vi "Visualize Puzzle.vi"(7 "Jump Points":set{T2}(c389), 10 "Direction Planes":T1[][][](array[typedef]), 11 "Wall Array":T1[][](array[typedef])) -> (3 "Array out":T1[][](array[typedef]))   [LabVIEW 2020]
uses:
  RB ENUM_Position ID.ctl
  Cluster _Point Location.ctl
  038fd235-bb71-4006-9680-315b02cd736b.vi
  <vilib>/Comparison/Equal/Equal Functor/Equal Functor.lvclass
panel:
  out "colum":i32
  out "row":i32
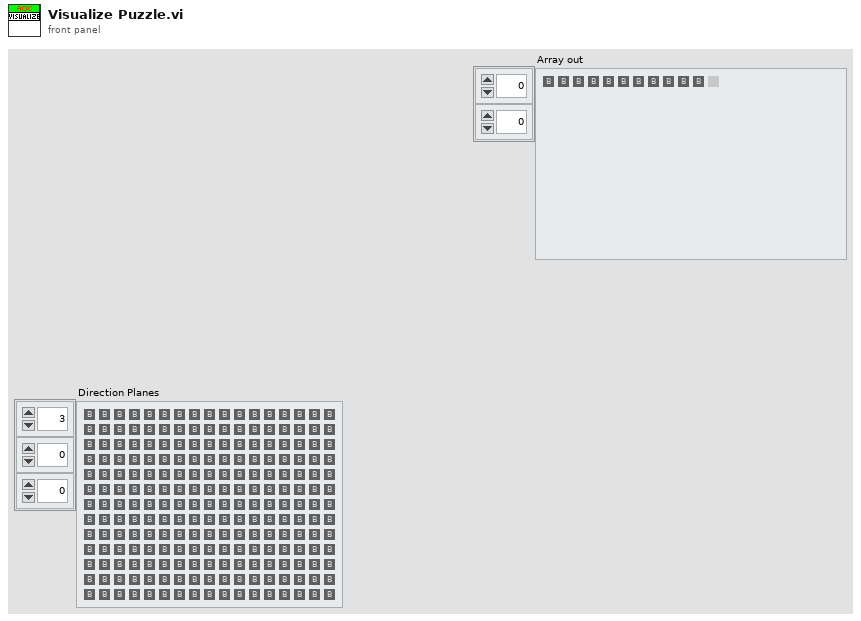
[diagram p1: front panel]
types:
  T1 = typedef "RB ENUM_Position ID.ctl" = enum32{"Blank", "Wall", "UP", "Down", "Left", "Right", "Two", "Three", "Four", "Spot"}
  T2 = typedef "Cluster _Point Location.ctl" = cluster{"X col":i32, "Y row":i32}
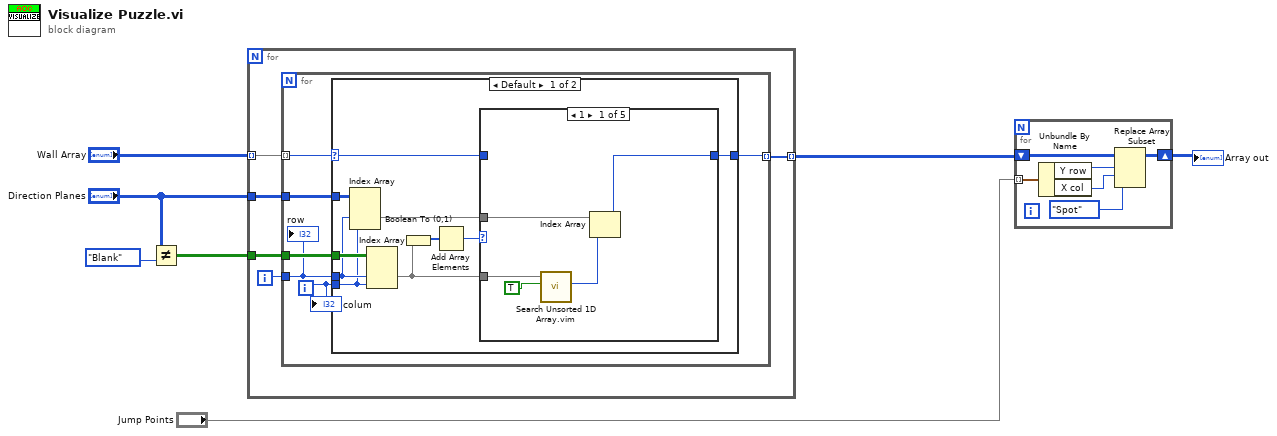
[diagram p0: block diagram]
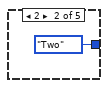
[diagram p2: hidden frame]
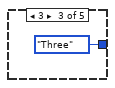
[diagram p3: hidden frame]
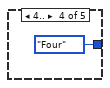
[diagram p4: hidden frame]
diagram:
  n1 = Not Equal?(x="Direction Planes", y=RB_ENUM_Position_ID."Blank" ("Position")) -> (x != y?=w1:bool[][][])
  n2 = for {
    tunnel: "Wall Array" -> [w12] mode=indexing
    tunnel: [w11] -> w4 mode=indexing
    tunnel: "Direction Planes" -> [w10]
    tunnel: w1 -> [w9]
    i -> [w8]
    n3 = for {
      tunnel: w12 -> [w18] mode=indexing
      tunnel: [w17] -> w11 mode=indexing
      tunnel: w10 -> [w13]
      tunnel: w9 -> [w16]
      tunnel: w8 -> [w15]
      i -> [w14]
      n4 = case shown="Default" w18 {
        selector: w18 -> [w24 w38]
        tunnel: [w23 w38] -> w17
        tunnel: w16 -> [w28 _]
        tunnel: w15 -> [w26 _]
        tunnel: w14 -> [w25 _]
        tunnel: w13 -> [w27 _]
        frame Default {
          n5 = Index Array(array=w27, index (dim 1)=w26, index (dim 2)=w25) -> (element=w22:T1[])  [unwired: 1 in]
          n6 = Index Array(array=w28, index (dim 1)=w26, index (dim 2)=w25) -> (element=w21:bool[])  [unwired: 1 in]
          n7 = Boolean To (0,1)(Boolean=w21) -> (0, 1=w19:i16[])
          n8 = Add Array Elements(numeric array=w19) -> (sum=w20:i16)
          n9 = case shown="1" w20 {
            tunnel: w24 -> [_ _ _ _ w37]
            tunnel: [w30 RB_ENUM_Position_ID."Two" ("Position") RB_ENUM_Position_ID."Three" ("Position") RB_ENUM_Position_ID."Four" ("Position") w37] -> w23
            tunnel: w22 -> [w31 _ _ _ _]
            tunnel: w21 -> [w33 _ _ _ _]
            frame 1 {
              n10 = call "Search Unsorted 1D Array.vim"("element"=TRUE, "unsorted 1D array"=w33) -> ("index of element"=w29:i32)  [unwired: 9 in]
              n11 = Index Array(array=w31, index=w29) -> (element=w30:T1)
            }
            frame 2 {
            }
            frame 3 {
            }
            frame 4.. {
            }
            frame ..0 {
            }
          }
        }
        frame "Wall" {
        }
      }
      "row" <- w15
      "colum" <- w14
    }
  }
  n12 = for {
    shift-right: [w43] -> w7
    shift-left: w4 -> [w44]
    tunnel: "Jump Points" -> [w42] mode=indexing
    n13 = Unbundle By Name(w42) -> ("Y row"=w41:i32, "X col"=w40:i32)
    n14 = Replace Array Subset(array=w44, new element=RB_ENUM_Position_ID."Spot" ("Position"), index (row)=w41, index (col)=w40) -> (w43:T1[][])
  }
  "Array out" <- w7
